vi "Pop Up.vi"(11 "Dev Actor in":refnum<class "Dev Actor.lvclass">) -> (3 "Dev Actor out":refnum<class "Dev Actor.lvclass">)   [LabVIEW 2021, in "Dev Actor.lvlib" / "Dev Actor.lvclass"]
uses:
  Dev Actor.lvclass
  C:/git/jettl/src/Actor/Actor/Actor.lvclass
  Dev Actor.lvclass/Dev Actor.ctl
  <vilib>/numeric/Random Number (Range) U64.vi
  <vilib>/numeric/sub_Random U32.vi
  Actor/Msgs/Create/Create Msg/Create Msg.lvclass
  C:/git/jettl/src/Actor/Msg/Msg.lvclass
  Dev Panel/Dev Panel.lvclass
  C:/git/jettl/src/Actor/Msgs/Create/Create/Create.lvclass
  C:/git/jettl/src/Actor/Msgs/Last Ack/Last Ack/Last Ack.lvclass
  C:/git/jettl/src/Actor/Msgs/Merge Error/Merge Error/Merge Error.lvclass
  C:/git/jettl/src/Actor/Msgs/Override Error/Override Error/Override Error.lvclass
  C:/git/jettl/src/Actor/Msgs/Teardown/Teardown/Teardown.lvclass
  C:/git/jettl/src/temp/Dev Actor/Dev Actor/Dev Actor.lvclass
  C:/git/jettl/src/temp/Msgs/Pop Up/Pop Up/Pop Up.lvclass
  C:/git/jettl/src/Actor/Msgs/Create/Create Msg/Create Msg.lvclass
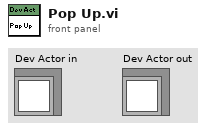
[diagram p1: front panel]
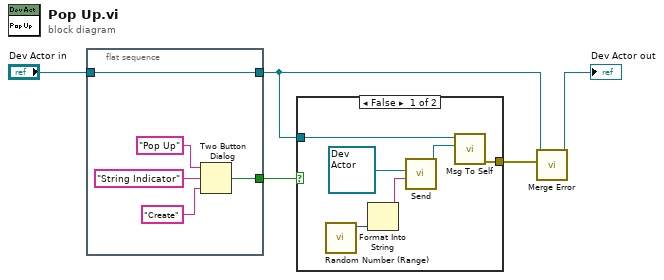
[diagram p0: block diagram]
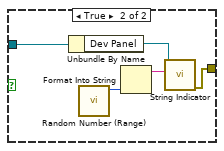
[diagram p2: hidden frame]
diagram:
  n1 = flat-sequence {
    tunnel: [w10] -> w1
    tunnel: "Dev Actor in" -> [w10]
    tunnel: [w7] -> w4
    frame #0 {
      n2 = Two Button Dialog(message="Pop Up", 1:"Create" ("F button name (\"Cancel\")"), 2:"String Indicator" ("T button name (\"OK\")")) -> (T button?=w7:bool)
    }
  }
  n3 = case shown="False" w4 {
    tunnel: w1 -> [w12 w21]
    tunnel: [w11 w17] -> w2
    frame False {
      n4 = call-poly <vilib>:"Random Number (Range).vi"() -> ("number"=w15:u64)  [unwired: 11 in]
      n5 = Format Into String(w15) -> (resulting string=w14:string)  [unwired: 3 in, 1 out]
      n6 = call "Send.vi"("Alias"=w14, "Actor"=refnum<class "Dev Actor.lvclass"> refnum ("Dev Actor.lvlib:Dev Actor.lvclass")) -> ("Create Msg out"=w13:refnum<class "Create Msg.lvclass">)  [unwired: 9 in]
      n7 = call-dynamic "Msg To Self.vi"("Msg"=w13, "Dev Actor in"=w12) -> ("error out"=w11:errorcluster)  [unwired: 9 in]
    }
    frame True {
      n8 = Unbundle By Name(w21) -> ("Dev Panel"=w20:refnum<class "Dev Panel.lvclass">)
      n9 = call-poly <vilib>:"Random Number (Range).vi"() -> ("number"=w19:u64)  [unwired: 11 in]
      n10 = Format Into String(w19) -> (resulting string=w18:string)  [unwired: 3 in, 1 out]
      n11 = call "String Indicator.vi"("String Indicator"=w18, "Dev Panel in"=w20) -> ("error out"=w17:errorcluster)  [unwired: 9 in]
    }
  }
  n12 = call-dynamic "Merge Error.vi"("Error"=w2, "Dev Actor in"=w1) -> ("Dev Actor out"=→"Dev Actor out":refnum<class "Dev Actor.lvclass">)  [unwired: 9 in]
